vi "Sensor Data.vi"   [LabVIEW 2015, in "Lake Shore 350.lvlib"]
uses:
  Lake Shore 350.lvlib
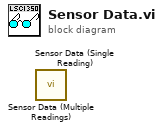
[diagram p0: block diagram]
diagram:
  n1 = call "Sensor Data (Multiple Readings).vi"() -> ()  [unwired: 9 in, 3 out]
  n2 = call "Sensor Data (Single Reading).vi"() -> ()  [unwired: 9 in, 3 out]
